vi "Initialize Tip Group.vi"(8 "error in (no error)":errorcluster, 11 "Refnum in":T1) -> (0 "error out":errorcluster, 3 "Refnum out":T1)   [LabVIEW 2020]
doc: "This VI initializes a group so that it is recognized by IMAQ."
uses:
  <vilib>/vision/Image Controls.llb/IMAQ Image.ctl
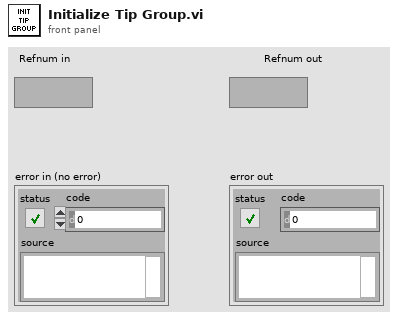
[diagram p1: front panel]
types:
  T1 = typedef "IMAQ Image.ctl" = refnum<image>
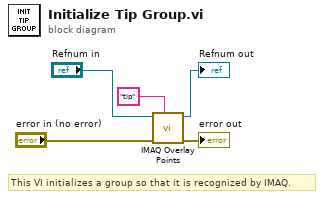
[diagram p0: block diagram]
diagram:
  # "This VI initializes a group so that it is recognized by IMAQ."
  n1 = call "IMAQ Overlay Points"("Group"="tip", "error in (no error)"="error in (no error)", "Image"="Refnum in") -> ("error out"=→"error out":errorcluster, "Image Out"=→"Refnum out":T1)  [unwired: 7 in]
